vi "Load PrefDialog For an INI File.vi"(8 "Error Array In":errorcluster[](array[cluster]), 10 "PathToPluginINI":path, 11 "Module Name":string="Sensor") -> (0 "ErrorArray Out":errorcluster[](array[cluster]))   [LabVIEW 2018]
uses:
  NistPluggableModules/TestClass/Test.lvclass
  NistPluggableModules/TestClass/Test.lvclass/Test.ctl
  NistPluggableModules/TestClass/Accessors/Read ModuleIDs.vi
  NistPluggableModules/TestClass/Accessors/Read ModuleList.vi
  <userlib>/NIST/NISTErrorLib/NISTErrorLib.lvlib
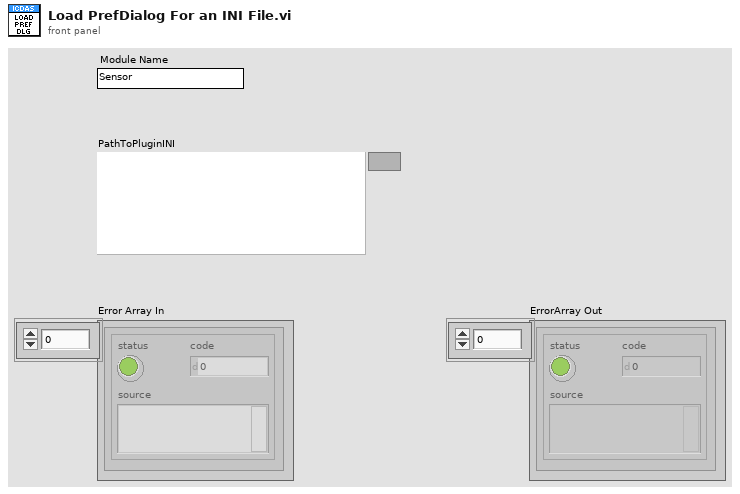
[diagram p1: front panel]
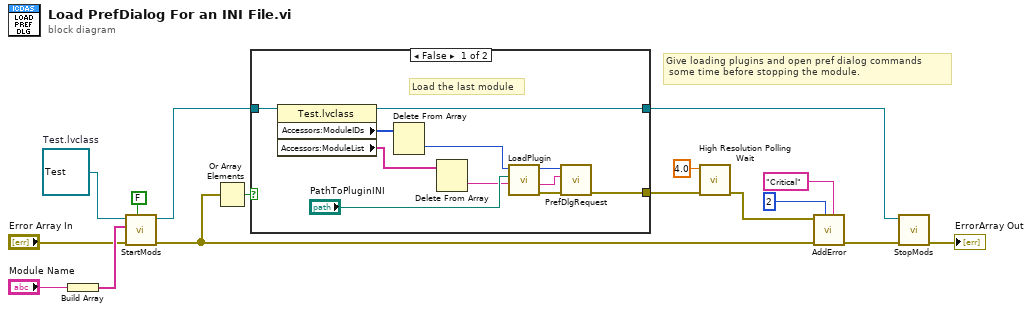
[diagram p0: block diagram]
diagram:
  w16 = refnum<class "Test.lvclass"> refnum  # Test.lvclass
  # "Give loading plugins and open pref dialog commands\n some time before stopping the module."
  n1 = Build Array("Module Name") -> (w10:string[])
  n2 = call "StartMods.vi"("ShowPanel? (f)"=FALSE, "Error Array In"="Error Array In", "Module List"=w10, "Test.lvclass"=w16) -> ("Error Array Out"=w3:errorcluster[], "Test.lvclass"=w13:refnum<class "Test.lvclass">)  [unwired: 5 in, 1 out]
  n3 = Or Array Elements(Boolean array=w3) -> (logical OR=w14:bool)
  n4 = case shown="False" w14 {
    tunnel: w13 -> [w27 w28]
    tunnel: [w26 w28] -> w12
    tunnel: [w19 _] -> w6
    frame False {
      # "Load the last module"
      n5 = property class="Test.lvclass"(reference=w27) -> (reference out=w26:refnum<class "Test.lvclass">, "Accessors:ModuleIDs"=w24:i32[], "Accessors:ModuleList"=w18:string[])  [unwired: 1 in, 1 out]
      n6 = Delete From Array(array=w24) -> (deleted portion=w23:i32)  [unwired: 2 in, 1 out]
      n7 = Delete From Array(array=w18) -> (deleted portion=w17:string)  [unwired: 2 in, 1 out]
      n8 = call "LoadPlugin.vi"("Module Name"=w17, "INI File Path"="PathToPluginINI", "Module ID"=w23) -> ("error out"=w22:errorcluster, "Module Name out"=w20:string, "Module ID out"=w21:i32)  [unwired: 5 in, 1 out]
      n9 = call "PrefDlgRequest.vi"("error in (no error)"=w22, "Module Name"=w20, "Module ID"=w21) -> ("error out"=w19:errorcluster)  [unwired: 8 in]
    }
    frame True {
    }
  }
  n10 = call <vilib>:"High Resolution Polling Wait.vi"("error in (no error)"=w6, "seconds to wait"=4.0) -> ("error out"=w5:errorcluster)  [unwired: 9 in]
  n11 = call <userlib>:"AddError.vi"("Severity"="Critical", "Priority"=u8 2, "ErrorArray In"=w3, "error in (no error)"=w5) -> ("ErrorArray Out"=w2:errorcluster[])  [unwired: 6 in, 1 out]
  n12 = call "StopMods.vi"("ErrorArray In"=w2, "Test.lvclass"=w12) -> ("ErrorArray Out"=→"ErrorArray Out":errorcluster[])  [unwired: 8 in, 1 out]
